vi "Create Multirate Filter.vi"() -> ()   [LabVIEW 2023]
doc: "Demonstrates how to use the DFD Build MRate Filter VI and the DFD Build CIC Filter VI to create a multirate filter.\n\nComplete the following steps to use this VI.\n1) Run the VI.\n2) Change <B>h(n)</B> on the FIR page.\n3) Observe the magnitude response.\n4) View the CIC page.\n5) Change the basic parameters, such as the <B>Filter Type</B>, <B>Number of Stages</B>, and <B>Differential Delay</B>, of the cascaded integrator comb (CIC) filter.\n6) Observe the magnitude response.\n7) Change the <B>Filtering Mode</B> and <B>Factor</B> to see the effect on the Frequency axis of the Magnitude Response graph.\n8) Click the <B>STOP</B> button to stop this VI.\n9) Examine the block diagram to learn how to create multirate filters."
uses:
  <vilib>/addons/Digital Filter Design/_Objects.llb/DFD Multirate Filtering Mode.ctl
  <vilib>/addons/Digital Filter Design/FilterLib.llb/DFD Build MRate Filter from TF.vi
  <vilib>/addons/Digital Filter Design/NI_DigFilterLicensed.lvlib
panel:
  in  "stop":bool
  out "Error Message":string
  out "Magnitude Response":cluster{"f0":dbl, "df":dbl, "values":dbl[]}[](graph)
  in  "Filtering Mode":T1=2 items=["No Rate Change", "Interpolation", "Decimation"]
  in  "Factor":i32=2
  in  "structure":enum32{"FIR", "CIC"}(tab)
  in  "h(n)":dbl[](array[numeric])=[0.5, 0.5]
  in  "Differential Delay":i32=2
  in  "Number of Stages":i32=2
  in  "Filter Type":enum16{"Lowpass", "Highpass"}(ring)
  # "Select Help>>Show Context Help and move the cursor over the VI icon for more information."
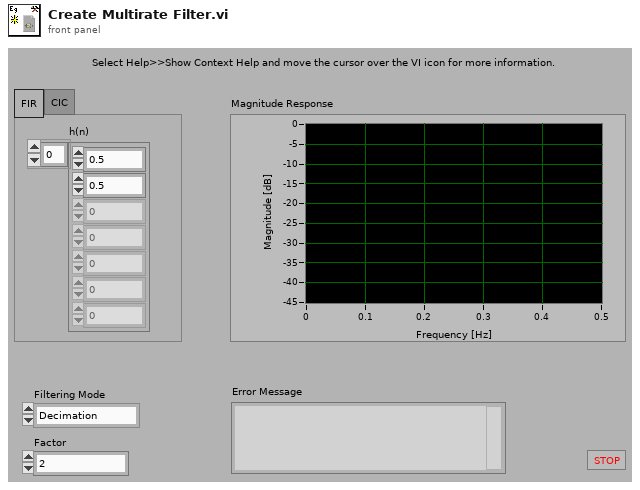
[diagram p1: front panel]
types:
  T1 = typedef "NI_DigFilterLicensed.lvlib/DFD Multirate Filtering Mode.ctl" = u16
  T2 = typedef "NI_DigFilterLicensed.lvlib/DFD Multirate Filter Obj.ctl" = cluster{"mMRate_Structure":enum16{"CIC", "FIR", "IIR", "Lattice"}, "mMRate_Mode":T3, "mMRate_Factor":i32, "mMRate_FIRParams":cluster{"mMRate_FIR_H":dbl[], "mMRate_FIR_IsNyquist?":bool, "mMRate_FIR_IsSymmetric?":bool}, "mMRate_CICParams":cluster{"mMRate_CIC_#Stage":i32, "mMRate_CIC_Lag":i32, "mMRate_CIC_Type":enum16{"Lowpass", "Highpass"}}, "mMRate_Order":i32, "mMRate_Version":string, "mMRate_Comments":string, "mMRate_RationalFactor":cluster{"mMRate_L":i32, "mMRate_M":i32}, "mMRate_Fs":dbl, "mMRate_Quantized?":bool, "mMRate_QFilterGain":dbl, "mMRate_CoefWl":i16, "mMRate_Scaling":cluster{"mMRate_ScaleByPowerOf2?":bool, "mMRate_ScaleType":T4}, "mMRate_InputWl":i16, "mMRate_OutputWl":i16, "mMRate_OutputMode":T5, "mMRate_MultMode":T6, "mMRate_BitPruning":bool, "mMRate_GainWl":i16, "mMRate_OutputFwl":i16, "mMRate_SumIwl":i16, "mMRate_InputIwl ":i16, "mMRate_SumWl":i16, "mMRate_CoefIwl":i16}
  T3 = typedef "NI_DigFilterLicensed.lvlib/DFD Multirate Mode.ctl" = i16
  T4 = typedef "NI_DigFilterLicensed.lvlib/DFD Coef Norm Type.ctl" = enum16{"No Norm", "Time Domain 1-Norm", "Time Domain 2-Norm", "Time Domain Inf-Norm"}
  T5 = typedef "NI_DigFilterLicensed.lvlib/DFD Round-off Mode.ctl" = enum16{"Nearest", "Truncation"}
  T6 = typedef "NI_DigFilterLicensed.lvlib/DFD FXP MRate Multiply Mode.ctl" = enum16{"Truncated", "Full"}
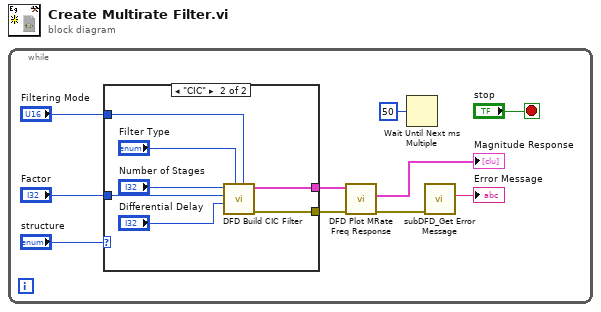
[diagram p0: block diagram]
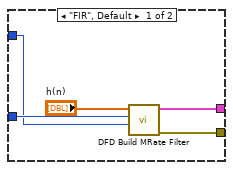
[diagram p2: hidden frame]
diagram:
  n1 = while {
    stop <- "stop" stop-if-true
    n2 = case shown="\"CIC\"" "structure" {
      tunnel: "Factor" -> [w14 w22]
      tunnel: "Filtering Mode" -> [w13 w21]
      tunnel: [w12 w18] -> w7
      tunnel: [w11 w17] -> w6
      frame "FIR", Default {
        n3 = call-poly <vilib>:"DFD Build MRate Filter.vi"("filtering mode"=w13, "factor"=w14, "h(n)"="h(n)") -> ("error out"=w11:errorcluster, "multirate filter out"=w12:T2)  [unwired: 2 in, 5 out]
      }
      frame "CIC" {
        n4 = call <vilib>:"DFD Build CIC Filter.vi"("filtering mode"=w21, "filter type"="Filter Type", "differential delay"="Differential Delay", "factor"=w22, "# stages"="Number of Stages") -> ("error out"=w17:errorcluster, "CIC filter out"=w18:T2)  [unwired: 2 in, 3 out]
      }
    }
    n5 = call <vilib>:"DFD Plot MRate Freq Response.vi"("error in (no error)"=w6, "multirate filter in"=w7) -> ("error out"=w3:errorcluster, "magnitude response"=→"Magnitude Response":cluster{"f0":dbl, "df":dbl, "values":dbl[]}[])  [unwired: 5 in, 3 out]
    n6 = Wait Until Next ms Multiple(millisecond multiple=u32 50) -> ()  [unwired: 1 out]
    n7 = call <vilib>:"subDFD_Get Error Message.vi"("error in (no error)"=w3) -> ("Error Message"=→"Error Message":string)  [unwired: 10 out]
  }
